vi "Auto2.vi"(0 "RobotDriveDevRef":T1, 11 "error in (no error)":errorcluster) -> (2 "Hook Center 2":dbl, 3 "Initial Hook Found 2":bool, 4 "Initial Hook Center 3":dbl, 6 "Pixels to turn 2":dbl, 8 "Initial Hook Center 6":dbl, 10 "Initial Hook Found 5":bool, 12 "Hook found 2":bool, 13 "Degrees to turn 2":dbl, 14 "Distance to wall (in) 2":dbl)   [LabVIEW 2016]
uses:
  <vilib>/Rock Robotics/WPI/RobotDrive/WPI_RobotDriveDevRef.ctl
  <vilib>/Rock Robotics/WPI/MotorControl/WPI_MotorControlDeviceRef.ctl
  <vilib>/Rock Robotics/WPI/MotorControl/WPI_MotorControlType.ctl
  <vilib>/Rock Robotics/SystemInterfaces/DIO/FPGA_DIOPWMChannel.ctl
  <vilib>/Rock Robotics/WPI/PWM/WPI_PWMDeadband.ctl
  <vilib>/Rock Robotics/WPI/RobotDrive/WPI_RobotDriveArcadeDrive_Standard(NoSaturation).vi
  Robot Global Data.vi
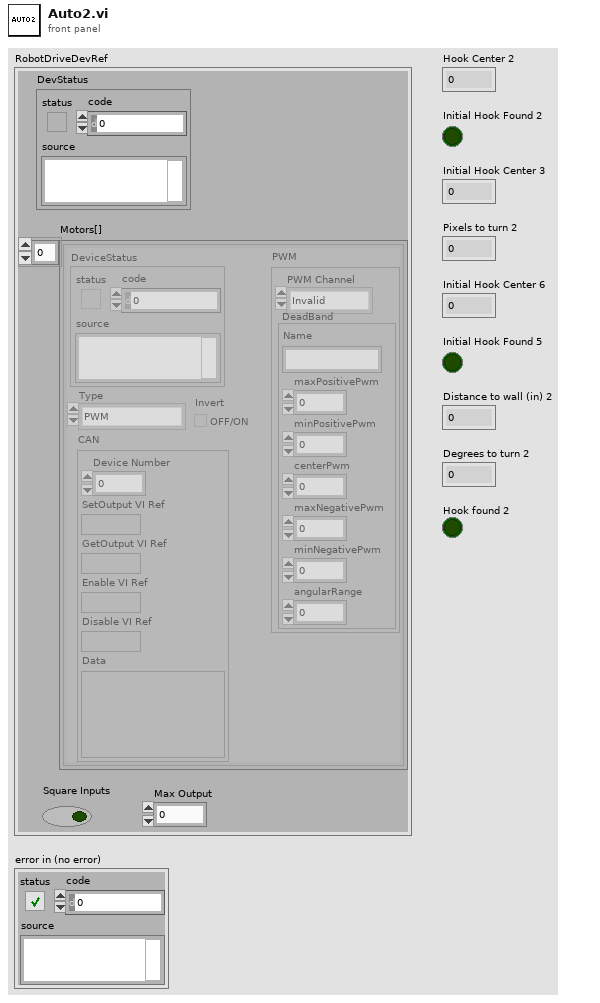
[diagram p1: front panel]
types:
  T1 = typedef "WPI_RobotDriveDevRef.ctl" = cluster{"DevStatus":errorcluster, "Motors[]":T2[], "Square Inputs":bool, "Max Output":dbl}
  T2 = typedef "WPI_MotorControlDeviceRef.ctl" = cluster{"DeviceStatus":errorcluster, "Type":T3, "PWM":cluster{"PWM Channel":T4, "DeadBand":T5}, "CAN":cluster{"Device Number":u8, "SetOutput VI Ref":variant, "GetOutput VI Ref":variant, "Enable VI Ref":variant, "Disable VI Ref":variant, "Data":variant}, "Invert":bool}
  T3 = typedef "WPI_MotorControlType.ctl" = enum16{"PWM", "CAN"}
  T4 = typedef "FPGA_DIOPWMChannel.ctl" = enum8{"PWM 0", "PWM 1", "PWM 2", "PWM 3", "PWM 4", "PWM 5", "PWM 6", "PWM 7", "PWM 8", "PWM 9", "PWM MXP 0", "PWM MXP 1", "PWM MXP 2", "PWM MXP 3", "PWM MXP 4", "PWM MXP 5", "PWM MXP 6", "PWM MXP 7", "PWM MXP 8", "PWM MXP 9", "Invalid"}
  T5 = typedef "WPI_PWMDeadband.ctl" = cluster{"Name":string, "maxPositivePwm":i32, "minPositivePwm":i32, "centerPwm":i32, "maxNegativePwm":i32, "minNegativePwm":i32, "angularRange":u16}
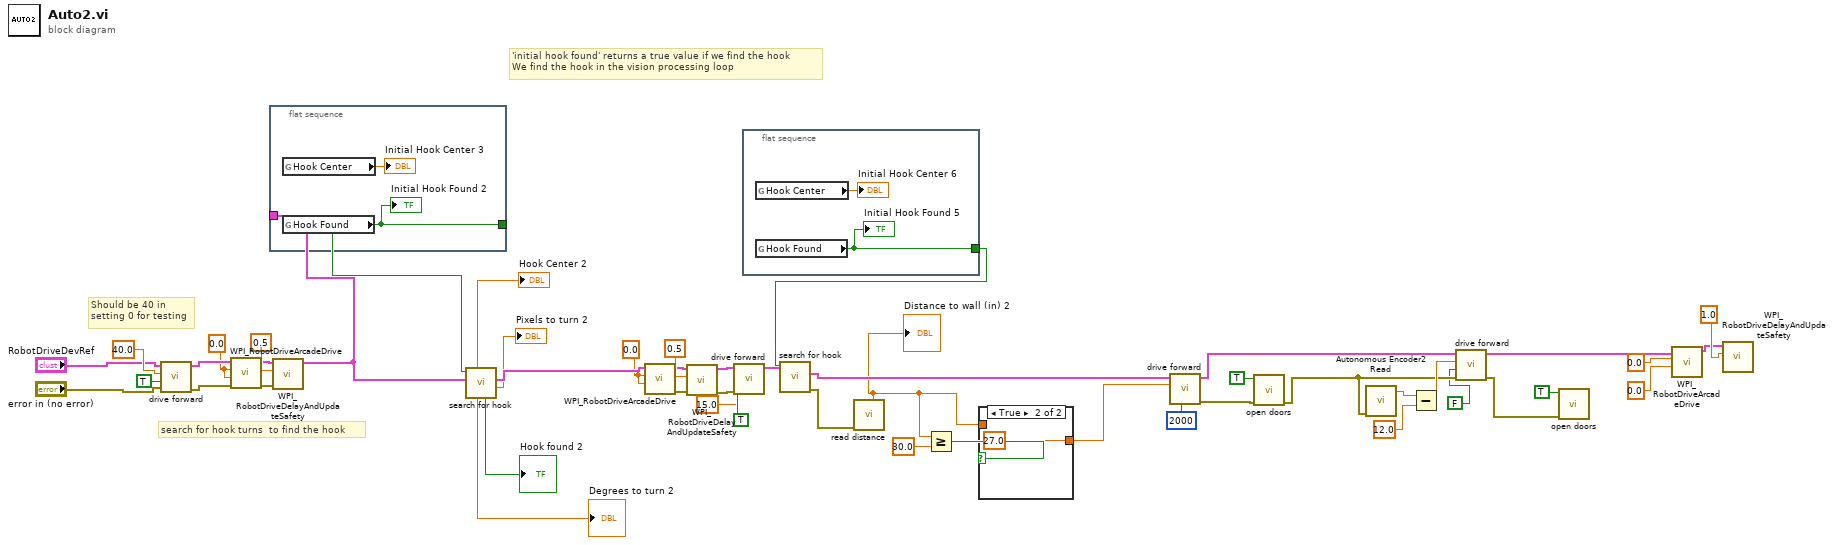
[diagram p0: block diagram]
diagram:
  w26 = 0.0 ("X axis value")
  w10 = 0.0 ("X axis value")
  # "'initial hook found' returns a true value if we find the hook \nWe find the hook in the vision processing loop"
  # "search for hook turns  to find the hook"
  # "Should be 40 in\nsetting 0 for testing"
  n1 = call "drive forward.vi"("error in (no error)"="error in (no error)", "forward"=TRUE, "desired distance"=40.0, "RobotDriveDevRef in"="RobotDriveDevRef") -> ("error out"=w12:errorcluster, "RobotDriveDevRef out"=w11:T1)  [unwired: 6 in]
  n2 = call-poly <vilib>:"WPI_RobotDriveArcadeDrive.vi"("error in (no error)"=w12, "Y axis value"=w10, "X axis value"=w10, "RobotDriveDevRef"=w11) -> ("error out"=w8:errorcluster, "RobotDriveDevRef"=w7:T1)  [unwired: 6 out]
  n3 = flat-sequence {
    tunnel: [w50] -> w14
    tunnel: w13 -> [_]
    frame #0 {
      n4 = global read "Robot Global Data.vi" "Hook Center"() -> (→"Initial Hook Center 3":dbl)
      n5 = global read "Robot Global Data.vi" "Hook Found"() -> (w50:bool)
      "Initial Hook Found 2" <- w50
    }
  }
  n6 = call <vilib>:"WPI_RobotDriveDelayAndUpdateSafety.vi"("error in (no error)"=w8, "Delay (s)"=0.5, "RobotDriveDevRef"=w7) -> ("RobotDriveDevRef 2"=w13:T1)  [unwired: 7 in, 1 out]
  n7 = call "search for hook.vi"("RobotDriveDevRef in"=w13, "Hook Found"=w14) -> ("Pixels to turn"=→"Pixels to turn 2":dbl, "RobotDriveDevRef out"=w27:T1, "Hook found"=→"Hook found 2":bool, "Degrees to turn"=→"Degrees to turn 2":dbl, "Hook Center"=→"Hook Center 2":dbl)  [unwired: 2 in, 3 out]
  n8 = call-poly <vilib>:"WPI_RobotDriveArcadeDrive.vi"("Y axis value"=w26, "X axis value"=w26, "RobotDriveDevRef"=w27) -> ("error out"=w24:errorcluster, "RobotDriveDevRef"=w23:T1)  [unwired: 1 in, 6 out]
  n9 = call <vilib>:"WPI_RobotDriveDelayAndUpdateSafety.vi"("error in (no error)"=w24, "Delay (s)"=0.5, "RobotDriveDevRef"=w23) -> ("error out"=w42:errorcluster, "RobotDriveDevRef 2"=w41:T1)  [unwired: 7 in]
  n10 = call "drive forward.vi"("error in (no error)"=w42, "forward"=TRUE, "desired distance"=15.0, "RobotDriveDevRef in"=w41) -> ("RobotDriveDevRef out"=w45:T1)  [unwired: 6 in, 1 out]
  n11 = flat-sequence {
    tunnel: [w52] -> w46
    frame #0 {
      n12 = global read "Robot Global Data.vi" "Hook Center"() -> (→"Initial Hook Center 6":dbl)
      n13 = global read "Robot Global Data.vi" "Hook Found"() -> (w52:bool)
      "Initial Hook Found 5" <- w52
    }
  }
  n14 = call "search for hook.vi"("RobotDriveDevRef in"=w45, "Hook Found"=w46) -> ("error out"=w48:errorcluster, "RobotDriveDevRef out"=w47:T1)  [unwired: 2 in, 6 out]
  n15 = call "read distance.vi"("error in (no error)"=w48) -> ("Distance 2"=w22:dbl)  [unwired: 9 in, 1 out]
  "Distance to wall (in) 2" <- w22
  n16 = Greater Or Equal?(x=w22, y=30.0) -> (x >= y?=w20:bool)
  n17 = case shown="True" w20 {
    tunnel: [w54 27.0 ("f")] -> w21
    tunnel: w22 -> [w54 _]
    frame False {
    }
    frame True {
    }
  }
  n18 = call "drive forward.vi"("time out"=2000, "desired distance"=w21, "RobotDriveDevRef in"=w47) -> ("error out"=w33:errorcluster, "RobotDriveDevRef out"=w34:T1)  [unwired: 7 in]
  n19 = call "open doors.vi"("error in (no error)"=w33, "Open"=TRUE) -> ("error out"=w37:errorcluster)  [unwired: 9 in]
  n20 = call "Autonomous Encoder2 Read.vi"("error in (no error)"=w37) -> ("Encoder Distance"=w38:dbl)  [unwired: 8 in, 2 out]
  n21 = Subtract(x=w38, y=12.0 ("desired distance")) -> (x-y=w39:dbl)
  n22 = call "drive forward.vi"("error in (no error)"=w37, "forward"=FALSE, "desired distance"=w39, "RobotDriveDevRef in"=w34) -> ("error out"=w1:errorcluster, "RobotDriveDevRef out"=w32:T1)  [unwired: 6 in]
  n23 = call "open doors.vi"("error in (no error)"=w1, "Open"=TRUE) -> ()  [unwired: 9 in, 1 out]
  n24 = call-poly <vilib>:"WPI_RobotDriveArcadeDrive.vi"("Y axis value"=0.0 ("X axis value"), "X axis value"=0.0, "RobotDriveDevRef"=w32) -> ("RobotDriveDevRef"=w30:T1)  [unwired: 1 in, 7 out]
  n25 = call <vilib>:"WPI_RobotDriveDelayAndUpdateSafety.vi"("Delay (s)"=1.0, "RobotDriveDevRef"=w30) -> ()  [unwired: 8 in, 2 out]
